vi "Help_VI_position.vi"(7 "Enum":T2(ring), 8 "Width-Height":cluster{"width":i16, "height":i16}, 11 "Bounds button":T1) -> (3 "Panel Bounds":T1={"Left"=200, "Top"=200, "Right"=500, "Bottom"=500})   [LabVIEW 2015]
uses:
  <vilib>/Utility/miscctls.llb/LVRectTypeDef.ctl
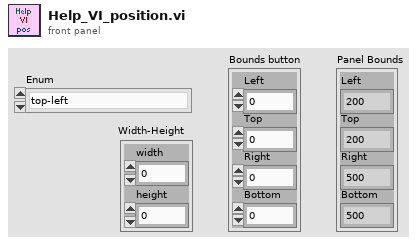
[diagram p1: front panel]
types:
  T1 = typedef "LVRectTypeDef.ctl" = cluster{"Left":i16, "Top":i16, "Right":i16, "Bottom":i16}
  T2 = enum16{"top-left", "top-right", "bot-left", "bot-right"}
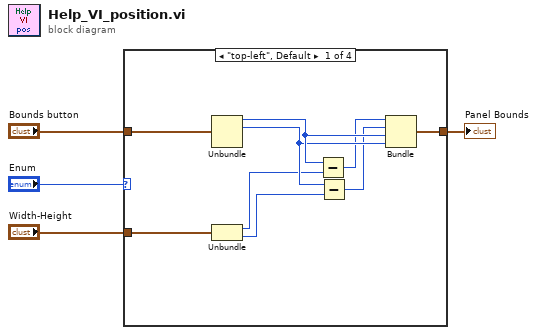
[diagram p0: block diagram]
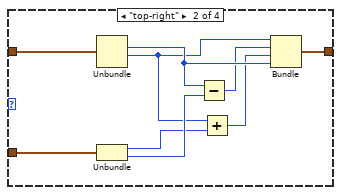
[diagram p2: hidden frame]
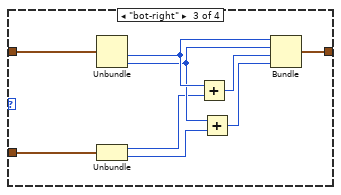
[diagram p3: hidden frame]
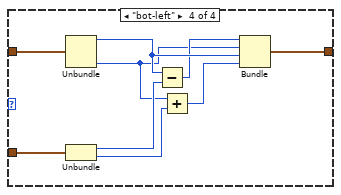
[diagram p4: hidden frame]
diagram:
  n1 = case shown="\"top-left\", Default" "Enum" {
    tunnel: "Bounds button" -> [w13 w22 w31 w40]
    tunnel: "Width-Height" -> [w12 w21 w30 w39]
    tunnel: [w5 w14 w29 w38] -> w1
    frame "top-left", Default {
      n2 = Unbundle(w13) -> ("Left"=w11:i16, "Top"=w10:i16)  [unwired: 2 out]
      n3 = Unbundle(w12) -> ("width"=w9:i16, "height"=w8:i16)
      n4 = Subtract(x=w11, y=w9) -> (x-y=w7:i16)
      n5 = Subtract(x=w10, y=w8) -> (x-y=w6:i16)
      n6 = Bundle(w7, w6, "Left"=w11, "Top"=w10) -> (w5:cluster{i16, i16, "Left":i16, "Top":i16})  [unwired: 1 in]
    }
    frame "top-right" {
      n7 = Unbundle(w22) -> ("Top"=w20:i16, "Right"=w17:i16)  [unwired: 2 out]
      n8 = Unbundle(w21) -> ("width"=w18:i16, "height"=w19:i16)
      n9 = Subtract(x=w20, y=w19) -> (x-y=w16:i16)
      n10 = Add(x=w17, y=w18) -> (x+y=w15:i16)
      n11 = Bundle("Right"=w17, w16, w15, "Top"=w20) -> (w14:cluster{"Right":i16, i16, i16, "Top":i16})  [unwired: 1 in]
    }
    frame "bot-right" {
      n12 = Unbundle(w31) -> ("Right"=w28:i16, "Bottom"=w27:i16)  [unwired: 2 out]
      n13 = Unbundle(w30) -> ("width"=w26:i16, "height"=w25:i16)
      n14 = Add(x=w28, y=w26) -> (x+y=w24:i16)
      n15 = Add(x=w27, y=w25) -> (x+y=w23:i16)
      n16 = Bundle("Right"=w28, "Bottom"=w27, w24, w23) -> (w29:cluster{"Right":i16, "Bottom":i16, i16, i16})  [unwired: 1 in]
    }
    frame "bot-left" {
      n17 = Unbundle(w40) -> ("Left"=w36:i16, "Bottom"=w34:i16)  [unwired: 2 out]
      n18 = Unbundle(w39) -> ("width"=w37:i16, "height"=w33:i16)
      n19 = Subtract(x=w36, y=w37) -> (x-y=w35:i16)
      n20 = Add(x=w34, y=w33) -> (x+y=w32:i16)
      n21 = Bundle(w35, "Bottom"=w34, "Left"=w36, w32) -> (w38:cluster{i16, "Bottom":i16, "Left":i16, i16})  [unwired: 1 in]
    }
  }
  "Panel Bounds" <- w1
